vi "HIOKI PW3390 Conf Interval.vi"(0 "VISA Resource":refnum<visa-resource-name>, 1 "Set/Query (F: Set)":bool, 5 "Interval (10: 1min)":T1(ring)=enum."1min", 11 "error in (no error)":errorcluster, 12 "OPC query (T: ON)":bool=TRUE, 13 "Error Out (F: Off)":bool) -> (4 "VISA Resource out":refnum<visa-resource-name>, 6 "Interval out":T1(ring)=enum."1min", 15 "error out":errorcluster)   [LabVIEW 2009]
doc: "Set/Query\n Set: Send the setting commands for the device.\n Query: Query the setting of the device.\n\nInterval\n Sets the Interval Time."
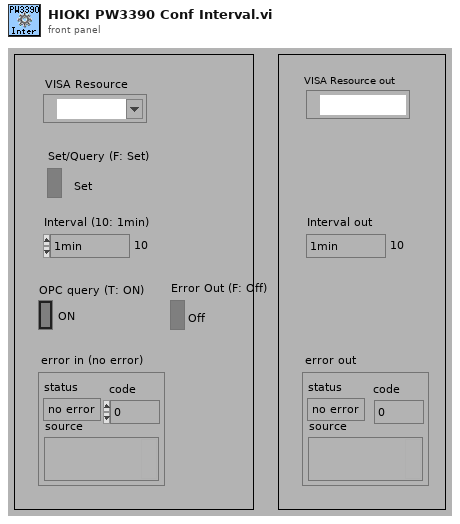
[diagram p1: front panel]
types:
  T1 = enum16{"OFF", "50ms", "100ms", "200ms", "500ms", "1s", "5s", "10s", "15s", "30s", "1min", "5min", "10min", "15min", "30min", "60min"}
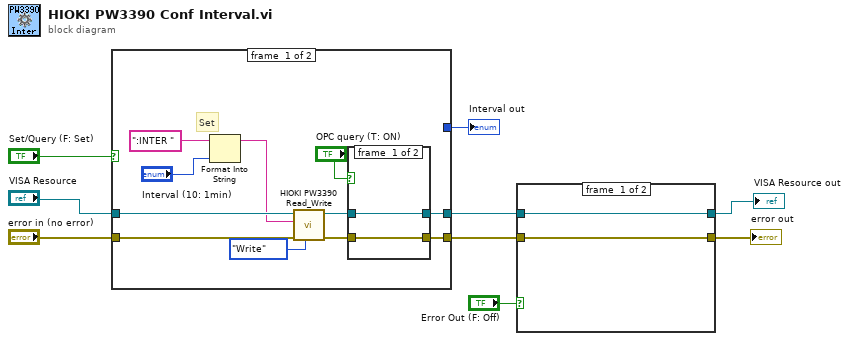
[diagram p0: block diagram]
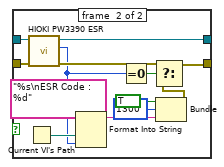
[diagram p2: hidden frame]
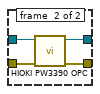
[diagram p3: hidden frame]
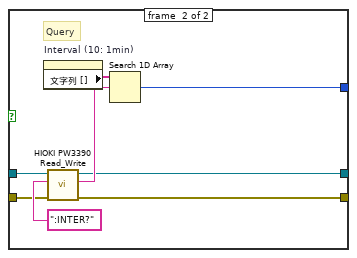
[diagram p4: hidden frame]
diagram:
  n1 = case shown="FALSE" "Set/Query (F: Set)" {
    tunnel: "error in (no error)" -> [w19 w33]
    tunnel: [w10 w28] -> w6
    tunnel: "VISA Resource" -> [w20 w32]
    tunnel: [w11 w27] -> w5
    tunnel: [_ w30] -> w3
    frame #0 {
      # "Set"
      n2 = Format Into String(initial string=":INTER ", "Interval (10: 1min)") -> (resulting string=w15:string)  [unwired: 2 in, 1 out]
      n3 = call <instrlib>:"HIOKI PW3390 Read_Write.vi"("Read/Write"=enum16{"Read", "Write"}."Write", "error in (no error)"=w19, "data in"=w15, "VISA Resource"=w20) -> ("error out"=w12:errorcluster, "VISA Resource out"=w13:refnum<visa-resource-name>)  [unwired: 5 in, 1 out]
      n4 = case shown="TRUE" "OPC query (T: ON)" {
        tunnel: [w22 w26] -> w11
        tunnel: [w21 w25] -> w10
        tunnel: w13 -> [w22 w24]
        tunnel: w12 -> [w21 w23]
        frame #0 {
        }
        frame #1 {
          n5 = call <instrlib>:"HIOKI PW3390 OPC.vi"("error in (no error)"=w23, "VISA Resource"=w24) -> ("error out"=w25:errorcluster, "VISA Resource out"=w26:refnum<visa-resource-name>)  [unwired: 7 in, 1 out]
        }
      }
    }
    frame #1 {
      # "Query"
      n6 = property on="Interval (10: 1min)" class="Enum (strict)"() -> ("文字列 []"=w29:string[])  [unwired: 2 in, 2 out]
      n7 = call <instrlib>:"HIOKI PW3390 Read_Write.vi"("error in (no error)"=w33, "data in"=":INTER?", "VISA Resource"=w32) -> ("error out"=w28:errorcluster, "data out"=w31:string, "VISA Resource out"=w27:refnum<visa-resource-name>)  [unwired: 6 in]
      n8 = Search 1D Array(1D array=w29, element=w31) -> (index of element=w30:i32)  [unwired: 1 in]
    }
  }
  "Interval out" <- w3
  n9 = case shown="TRUE" "Error Out (F: Off)" {
    tunnel: w5 -> [w36 w49]
    tunnel: w6 -> [w35 w48]
    tunnel: [w35 w38] -> w4
    tunnel: [w36 w47] -> w1
    frame #0 {
    }
    frame #1 {
      n10 = Current VI's Path() -> (path=w45:path)
      n11 = call <instrlib>:"HIOKI PW3390 ESR.vi"("error in (no error)"=w48, "VISA Resource"=w49) -> ("error out"=w39:errorcluster, "Output Value"=w37:u8, "VISA Resource out"=w47:refnum<visa-resource-name>)  [unwired: 6 in, 1 out]
      n12 = Format Into String(format string="%s\nESR Code : %d", w45, w37) -> (resulting string=w41:string)  [unwired: 2 in, 1 out]
      n13 = Equal To 0?(x=w37) -> (x = 0?=w46:bool)
      n14 = Bundle("status"=TRUE, "code"=1300, w41) -> (w40:cluster{"status":bool, "code":i32, string})  [unwired: 1 in]
      n15 = Select(t=w39, s=w46, f=w40) -> (s? t:f=w38:errorcluster)
    }
  }
  "error out" <- w4
  "VISA Resource out" <- w1
